vi "RT Driver VI.vi"(7 "Operation":T1, 11 "Device Reference in":T2 format="%.0x") -> (0 "Error Code":i32)   [LabVIEW 2015, in "Protection and Rolling Counter Addon Engine.lvlib"]
uses:
  Protection and Rolling Counter Addon Engine.lvlib
  <vilib>/NI Veristand/Custom Device API/Custom Device Item Ref.ctl
  <vilib>/NI Veristand/Custom Device API/Hardware Interface Driver VI Operation.ctl
  <vilib>/NI/NIVS Inline Async API/_VS Inline Async API/VS Inline Async API/VS Inline Async API.lvclass
  Types/RT Async Engine Variables.ctl
  Types/RT Frame Settings.ctl
  Types/RT Protection Configuration.ctl
  Shared/Types/Protection Type.ctl
  Shared/Types/InputChannelConfiguration.ctl
  Types/RT Counter Settings.ctl
  Shared/Types/Exported.OnCompile.ctl
  Shared/Types/XNET Settings.ctl
  Shared/Types/Exported Frame Settings.ctl
  Shared/Types/Exported Protection Settings.ctl
  Shared/Types/Exported Counter Settings.ctl
  <vilib>/NI/NIVS Inline Async API/_VS Inline Async API/VS Inline Async API/VS Inline Async API.lvclass/VS Inline Async API.ctl
  <vilib>/NI/NIVS Inline Async API/_Data Access Engine/Data Access Engine/Data Access Engine.lvclass/Data Access Engine.ctl
  <vilib>/NI/NIVS Inline Async API/_Data Access Engine/Access Type Classes/Write/Write.lvclass/Write.ctl
  <vilib>/NI/NIVS Inline Async API/_Data Access Engine/Access Type Classes/ReadWrite/ReadWrite.lvclass/ReadWrite.ctl
  <vilib>/NI/NIVS Inline Async API/_Data Access Engine/Access Type Classes/Read/Read.lvclass/Read.ctl
  <vilib>/NI/NIVS Inline Async API/_Data Access Engine/Data Access Engine/Methods/Data.Engine.Read Data from HW.vi
  <vilib>/NI/NIVS Inline Async API/_VS Inline Async API/Error Handling Process/SubVIs/Error.GetError.vi
  <vilib>/NI/NIVS Inline Async API/_Data Access Engine/Data Access Engine/Methods/Data.Engine.Write Data to HW.vi
  <vilib>/NI/NIVS Inline Async API/_Data Access Engine/Access Type Classes/ReadWrite/ReadWrite.EngineData.vi
  <vilib>/NI/NIVS Inline Async API/_Data Access Engine/Access Type Classes/Write/Write.EngineData.vi
  <vilib>/NI/NIVS Inline Async API/_Data Access Engine/Access Type Classes/Read/Read.EngineData.vi
  <vilib>/NI Veristand/Custom Device API/NI VeriStand - Get Channel Value by Data Reference.vi
  <vilib>/NI Veristand/Custom Device API/NI VeriStand - Set Channel Value by Data Reference.vi
  <vilib>/NI Veristand/Custom Device API/NI VeriStand - Get Channel Values by Block Data Reference.vi
  Shared/SubVIs/GUID Lookup.vi
  <vilib>/NI Veristand/Custom Device API/Get Item Property (Variant).vi
  <vilib>/NI Veristand/Custom Device API/Global Data Refs.vi
  <vilib>/NI VeriStand/Custom Device Tools/Custom Device Utility Library/Custom Device Utility Library.lvlib
  <vilib>/NI VeriStand/Custom Device API/Custom Device API.lvlib
  Shared/Protection and Rolling Counter Addon Shared.lvlib
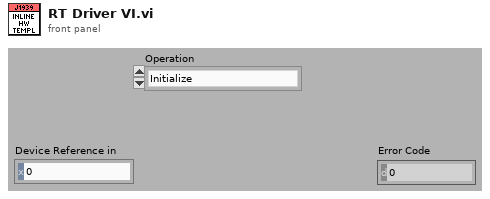
[diagram p1: front panel]
types:
  T1 = typedef "Custom Device API.lvlib/Hardware Interface Driver VI Operation.ctl" = enum16{"Initialize", "Start", "Read Data from HW", "Write Data to HW", "Close"}
  T2 = typedef "Custom Device API.lvlib/Custom Device Item Ref.ctl" = u64
  T3 = typedef "Protection and Rolling Counter Addon Engine.lvlib/RT Async Engine Variables.ctl" = cluster{"Priority":i32, "CAN Session":refnum<k21>, "Frame Count":i32, "Frames":T4[]}
  T4 = typedef "Protection and Rolling Counter Addon Engine.lvlib/RT Frame Settings.ctl" = cluster{"Frame ID":u32, "Payload Length":u32, "VS Offset":i32, "VS Length":i32, "Frame Conversion":refnum<k21>, "Frame.PrevData":dbl[], "Generation Period":u32, "Time Since Last Generation":u32, "Generation Iterations":u32, "Generation Counter":u32, "Has Protection?":bool, "Protection Configurations":T5[], "Has Counter":bool, "Counter Configurations":T8[], "Has Disable?":bool, "Disable VS Index":i32}
  T5 = typedef "Protection and Rolling Counter Addon Engine.lvlib/RT Protection Configuration.ctl" = cluster{"Protection Frame Index":i32, "Protection Type":T6, "Data Indeces":i32[], "Initialized Data Array":dbl[], "Check Sum Conversion":refnum<k21>, "CRC Channels":T7[], "Protection VS Index":i32}
  T6 = typedef "Protection and Rolling Counter Addon Shared.lvlib/Protection Type.ctl" = enum16{"Arb ID + Bytes Checksum with Inversion", "Arb ID + Bytes CRC with Inversion", "Reversed Raw Signal Checksum with Inversion"}
  T7 = typedef "Protection and Rolling Counter Addon Shared.lvlib/InputChannelConfiguration.ctl" = cluster{"Start Bit":i32, "Name":string, "Number of bits":i32, "Scale":dbl, "Offset":dbl, "Data Type":u32}
  T8 = typedef "Protection and Rolling Counter Addon Engine.lvlib/RT Counter Settings.ctl" = cluster{"Counter Frame Index":i32, "Max Count":dbl, "Counter VS Index":i32}
  T9 = cluster{"Process":refnum<class "VS Inline Async API.lvclass">, "Device.Error":errorcluster, "RT Configuration":T3}
  T10 = typedef "Protection and Rolling Counter Addon Shared.lvlib/Exported.OnCompile.ctl" = cluster{"XNET Settings":T11, "Frames":T12[]}
  T11 = typedef "Protection and Rolling Counter Addon Shared.lvlib/XNET Settings.ctl" = cluster{"Database":refnum<k21>, "Cluster":refnum<k21>, "Port":string, "Baud rate [Bd]":u64, "Termination":u32, "CAN I/O Mode":u32, "FD Baud rate [Bd]":u64, "Priority":i32, "Use Legacy":bool}
  T12 = typedef "Protection and Rolling Counter Addon Shared.lvlib/Exported Frame Settings.ctl" = cluster{"Frame ID":u32, "Payload Length":u32, "Signal XNET Paths":string[], "VS Offset":i32, "VS Length":i32, "Generation Period":u32, "Has Protection?":bool, "Protection Configurations":T13[], "Has Counter":bool, "Counter Configurations":T14[], "Has Disable?":bool, "Disable VS Index":i32, "Frame.PrevData":dbl[]}
  T13 = typedef "Protection and Rolling Counter Addon Shared.lvlib/Exported Protection Settings.ctl" = cluster{"Protection Frame Index":i32, "Protection Type":T6, "Data Indeces":i32[], "Initialized Data Array":dbl[], "Protection Signal XNET Paths":string[], "CRC Channels":T7[], "Protection VS Update Index":i32}
  T14 = typedef "Protection and Rolling Counter Addon Shared.lvlib/Exported Counter Settings.ctl" = cluster{"Counter Frame Index":i32, "Max Count":dbl, "Counter VS Index":i32}
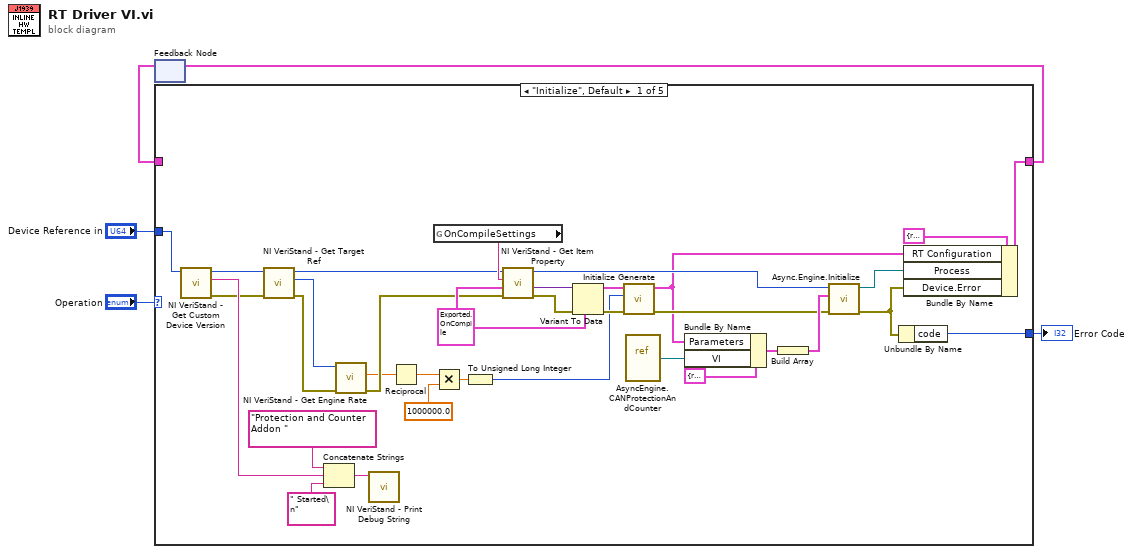
[diagram p0: block diagram]
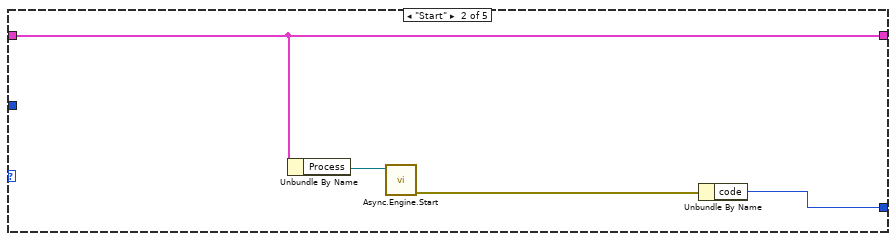
[diagram p2: hidden frame]
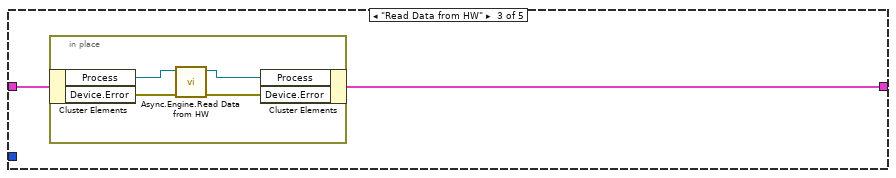
[diagram p3: hidden frame]
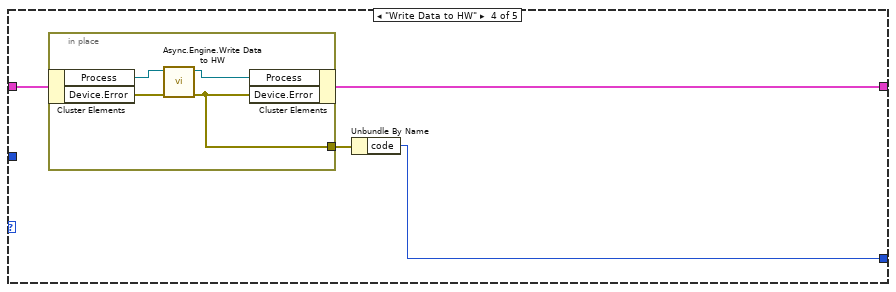
[diagram p4: hidden frame]
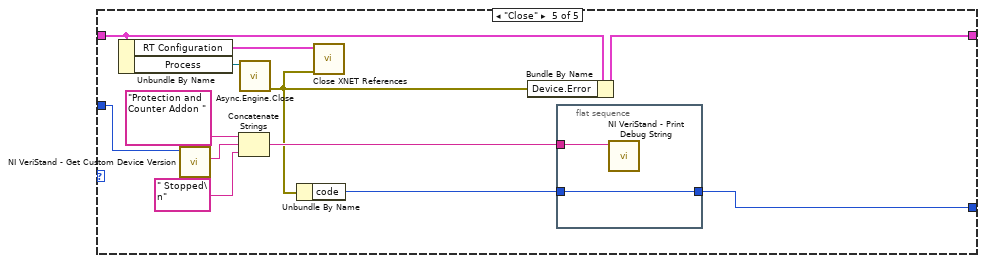
[diagram p5: hidden frame]
diagram:
  n1 = feedback #1() -> (w3:T9)  [unwired: 1 out]
  n2 = case shown="\"Initialize\", Default" "Operation" {
    tunnel: [w38 w40 w44 w53 w69] -> w4
    tunnel: w3 -> [_ w40 w45 w52 w61]
    tunnel: [w39 w43 _ w50 w62] -> w2
    tunnel: "Device Reference in" -> [w35 _ _ _ w65]
    frame "Initialize", Default {
      w22 = T10 {"XNET Settings"={"Database"="", "Cluster"="", "Port"="", "Baud rate [Bd]"=500000, "Termination"=1, "CAN I/O Mode"=0, "FD Baud rate [Bd]"=500000, "Priority"=100, "Use Legacy"=FALSE}, "Frames"=[]} ("Cluster")
      n3 = call <vilib>:"NI VeriStand - Get Custom Device Version.vi"("Device Ref in"=w35) -> ("error out"=w14:errorcluster, "Value"=w34:string, "Device Ref out"=w25:T2)  [unwired: 8 in]
      n4 = call <vilib>:"NI VeriStand - Get Target Ref.vi"("error in"=w14, "Item Ref in"=w25) -> ("error out"=w13:errorcluster, "Target Ref"=w15:T2, "Item Ref out"=w16:T2)  [unwired: 6 in, 1 out]
      n5 = Concatenate Strings("Protection and Counter Addon " ("Debug String"), w34, " Started\n" ("string")) -> (w36:string)
      n6 = call <vilib>:"NI VeriStand - Get Engine Rate.vi"("error in (no error)"=w13, "Item Ref in"=w15) -> ("error out"=w12:errorcluster, "Rate (Hz)"=w11:dbl)  [unwired: 7 in, 1 out]
      n7 = call <vilib>:"NI VeriStand - Print Debug String.vi"("Message"=w36) -> ()  [unwired: 10 in, 1 out]
      n8 = Reciprocal(x=w11) -> (1/x=w10:dbl)
      n9 = global read "GUID Lookup.vi" "OnCompileSettings"() -> (w26:string)
      n10 = Multiply(x=w10, y=1000000.0) -> (x*y=w8:dbl)
      n11 = To Unsigned Long Integer(number=w8) -> (unsigned 32bit integer=w7:u32)
      n12 = call-poly <vilib>:"NI VeriStand - Get Item Property.vi"("error in (no error)"=w12, "Default Value"=w22, "Property Name"=w26, "Item Ref in"=w16) -> ("error out"=w23:errorcluster, "Value"=w24:variant, "Item Ref out"=w21:T2)  [unwired: 4 in, 1 out]
      n13 = Variant To Data(error in=w23, type=w22, Variant=w24) -> (data=w18:T10, error out=w20:errorcluster)
      n14 = call "Initialize Generate.vi"("error in (no error)"=w20, "PCL (usec)"=w7, "OnCompile Variables"=w18) -> ("error out"=w19:errorcluster, "RT Configuration"=w6:T3)  [unwired: 7 in]
      n15 = vi-ref "AsyncEngine.CANProtectionAndCounter.vi"() -> (w17:refnum<vi>)
      n16 = Bundle By Name(cluster=cluster{"VI":refnum<vi>, "Parameters":variant} {"VI"=refnum, "Parameters"=variant} ("Process"), "Parameters"=w6, "VI"=w17) -> (w29:cluster{"VI":refnum<vi>, "Parameters":variant})
      n17 = Build Array(w29) -> (w28:cluster{"VI":refnum<vi>, "Parameters":variant}[])
      n18 = call <vilib>:"Async.Engine.Initialize.vi"("error in (no error)"=w19, "Processes"=w28, "Custom Device Ref"=w21) -> ("error out"=w32:errorcluster, "Async"=w31:refnum<class "VS Inline Async API.lvclass">)  [unwired: 7 in]
      n19 = Unbundle By Name(w32) -> ("code"=w39:i32)
      n20 = Bundle By Name(cluster=T9 {"Process"=refnum, "Device.Error"={"status"=FALSE, "code"=0, "source"=""}, "RT Configuration"={"Priority"=100, "CAN Session"="", "Frame Count"=0, "Frames"=[]}} ("input cluster"), "RT Configuration"=w6, "Process"=w31, "Device.Error"=w32) -> (w38:T9)
    }
    frame "Start" {
      n21 = Unbundle By Name(w40) -> ("Process"=w42:refnum<class "VS Inline Async API.lvclass">)
      n22 = call <vilib>:"Async.Engine.Start.vi"("VS Inline Async API in"=w42) -> ("error out"=w41:errorcluster)  [unwired: 9 in, 1 out]
      n23 = Unbundle By Name(w41) -> ("code"=w43:i32)
    }
    frame "Read Data from HW" {
      n24 = in-place {
        n25 = in-place-cluster #2(w45) -> ("Process"=w49:refnum<class "VS Inline Async API.lvclass">, "Device.Error"=w47:errorcluster)
        n26 = call <vilib>:"Async.Engine.Read Data from HW.vi"("error in"=w47, "Async in"=w49) -> ("error out"=w46:errorcluster, "Async out"=w48:refnum<class "VS Inline Async API.lvclass">)  [unwired: 8 in]
        n27 = in-place-cluster #2("Process"=w48, "Device.Error"=w46) -> (w44:T9)
      }
    }
    frame "Write Data to HW" {
      n28 = in-place {
        in-place-border: [w54] -> w51
        n29 = in-place-cluster #3(w52) -> ("Process"=w56:refnum<class "VS Inline Async API.lvclass">, "Device.Error"=w57:errorcluster)
        n30 = call <vilib>:"Async.Engine.Write Data to HW.vi"("error in (no error)"=w57, "VS Inline Async API in"=w56) -> ("error out"=w54:errorcluster, "VS Inline Async API out"=w55:refnum<class "VS Inline Async API.lvclass">)  [unwired: 8 in]
        n31 = in-place-cluster #3("Process"=w55, "Device.Error"=w54) -> (w53:T9)
      }
      n32 = Unbundle By Name(w51) -> ("code"=w50:i32)
    }
    frame "Close" {
      n33 = Unbundle By Name(w61) -> ("RT Configuration"=w59:T3, "Process"=w60:refnum<class "VS Inline Async API.lvclass">)
      n34 = call <vilib>:"NI VeriStand - Get Custom Device Version.vi"("Device Ref in"=w65) -> ("Value"=w68:string)  [unwired: 8 in, 2 out]
      n35 = Concatenate Strings("Protection and Counter Addon " ("Debug String"), w68, " Stopped\n" ("Debug String")) -> (w64:string)
      n36 = call <vilib>:"Async.Engine.Close.vi"("Async in"=w60) -> ("error out"=w58:errorcluster)  [unwired: 9 in, 1 out]
      n37 = Unbundle By Name(w58) -> ("code"=w63:i32)
      n38 = call "Close XNET References.vi"("error in (no error)"=w58, "RT Configuration"=w59) -> ()  [unwired: 9 in, 1 out]
      n39 = Bundle By Name(cluster=w61, "Device.Error"=w58) -> (w69:T9)
      n40 = flat-sequence {
        tunnel: w64 -> [w71]
        tunnel: [w70] -> w62
        tunnel: w63 -> [w70]
        frame #0 {
          n41 = call <vilib>:"NI VeriStand - Print Debug String.vi"("Message"=w71) -> ()  [unwired: 10 in, 1 out]
        }
      }
    }
  }
  "Error Code" <- w2
  n42 = feedback-in #1(w4) -> ()
